vi "monedas denominacion.vi"(10 "Array":dbl[](array[numeric]), 11 "numero de ciclos":i32) -> (0 "Monedas de 10":dbl, 1 "Monedas de 5":dbl, 2 "Monedas de 2":dbl, 3 "Monedas de 1":dbl)   [LabVIEW 2019]
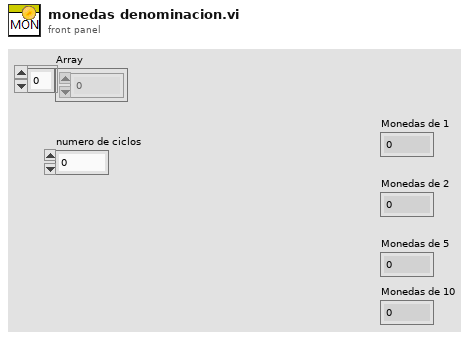
[diagram p1: front panel]
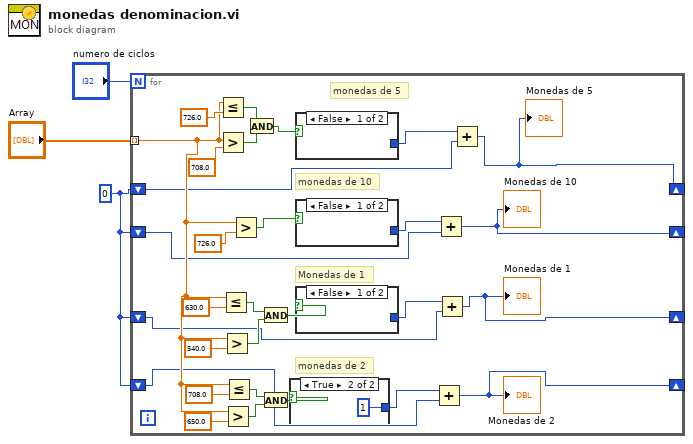
[diagram p0: block diagram]
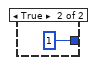
[diagram p3: hidden frame]
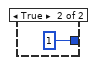
[diagram p4: hidden frame]
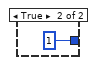
[diagram p5: hidden frame]
diagram:
  w1 = 0
  n1 = for {
    N: "numero de ciclos" -> [_]
    tunnel: "Array" -> [w21] mode=indexing
    shift-right: [w14] -> _
    shift-left: w1 -> [w13]
    shift-right: [w11] -> _
    shift-left: w1 -> [w10]
    shift-right: [w8] -> _
    shift-left: w1 -> [w7]
    shift-right: [w5] -> _
    shift-left: w1 -> [w4]
    # "monedas de 5"
    # "monedas de 10"
    # "monedas de 2"
    # "Monedas de 1"
    n2 = Less Or Equal?(x=w21, y=726.0 ("x")) -> (x <= y?=w31:bool)
    n3 = Greater?(x=w21, y=708.0) -> (0:w32:bool)
    n4 = Less Or Equal?(x=w21, y=630.0) -> (x <= y?=w24:bool)
    n5 = Greater?(x=w21, y=540.0) -> (0:w23:bool)
    n6 = Greater?(x=w21, y=650.0) -> (0:w17:bool)
    n7 = Less Or Equal?(x=w21, y=708.0) -> (x <= y?=w18:bool)
    n8 = Greater?(x=w21, y=726.0) -> (0:w27:bool)
    n9 = And(x=w31, y=w32) -> (x .and. y?=w30:bool)
    n10 = And(x=w24, y=w23) -> (x .and. y?=w22:bool)
    n11 = And(x=w18, y=w17) -> (x .and. y?=w16:bool)
    n12 = case shown="True" w16 {
      tunnel: [_ 1] -> w6
      frame False {
      }
      frame True {
      }
    }
    n13 = case shown="False" w30 {
      tunnel: [_ 1] -> w15
      frame False {
      }
      frame True {
      }
    }
    n14 = case shown="False" w27 {
      tunnel: [_ 1] -> w12
      frame False {
      }
      frame True {
      }
    }
    n15 = case shown="False" w22 {
      tunnel: [_ 1] -> w9
      frame False {
      }
      frame True {
      }
    }
    n16 = Add(x=w6, y=w4) -> (x+y=w5:i32)
    "Monedas de 2" <- w5
    n17 = Add(x=w12, y=w10) -> (x+y=w11:i32)
    "Monedas de 10" <- w11
    n18 = Add(x=w9, y=w7) -> (x+y=w8:i32)
    "Monedas de 1" <- w8
    n19 = Add(x=w15, y=w13) -> (x+y=w14:i32)
    "Monedas de 5" <- w14
  }
